vi "INI.GetPara.vi"(7 "section":string caption="Section", 8 "error in (no error)":errorcluster caption="错误输入（无错误）", 10 "Spec_name":string, 11 "INI_File":path) -> (0 "error out":errorcluster, 2 "Para out":string, 3 "ok?":bool)   [LabVIEW 2012, in "Lib_UEL.ATE.lvlib" / "Lib_App.lvlib"]
uses:
  Lib_App.lvlib
  <vilib>/Utility/config.llb/Read Key (String).vi
  <vilib>/Utility/config.llb/NI_LVConfig.lvlib
panel:
  # "说明:\n- 从配置文件读取参数."
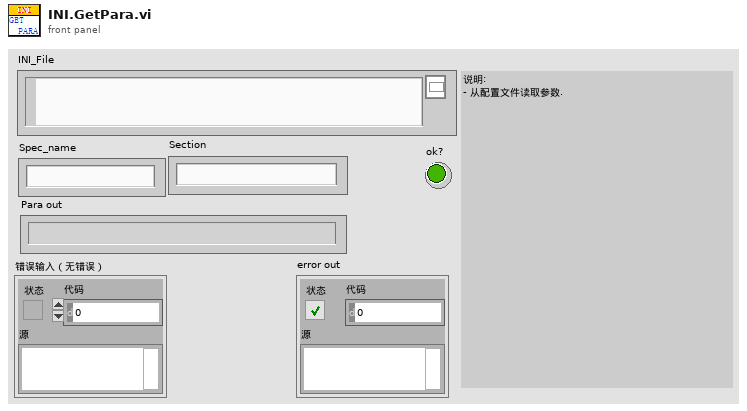
[diagram p1: front panel]
types:
  T1 = typedef "NI_LVConfig.lvlib/Config Data RefNum.ctl" = refnum<k1>
  T2 = cluster{"Item":string, "Unit":string, "Ref_value":dbl, "Low_limit_prod":dbl, "High_limit_prod":dbl, "Low_limit_qa":dbl, "High_limit_qa":dbl}
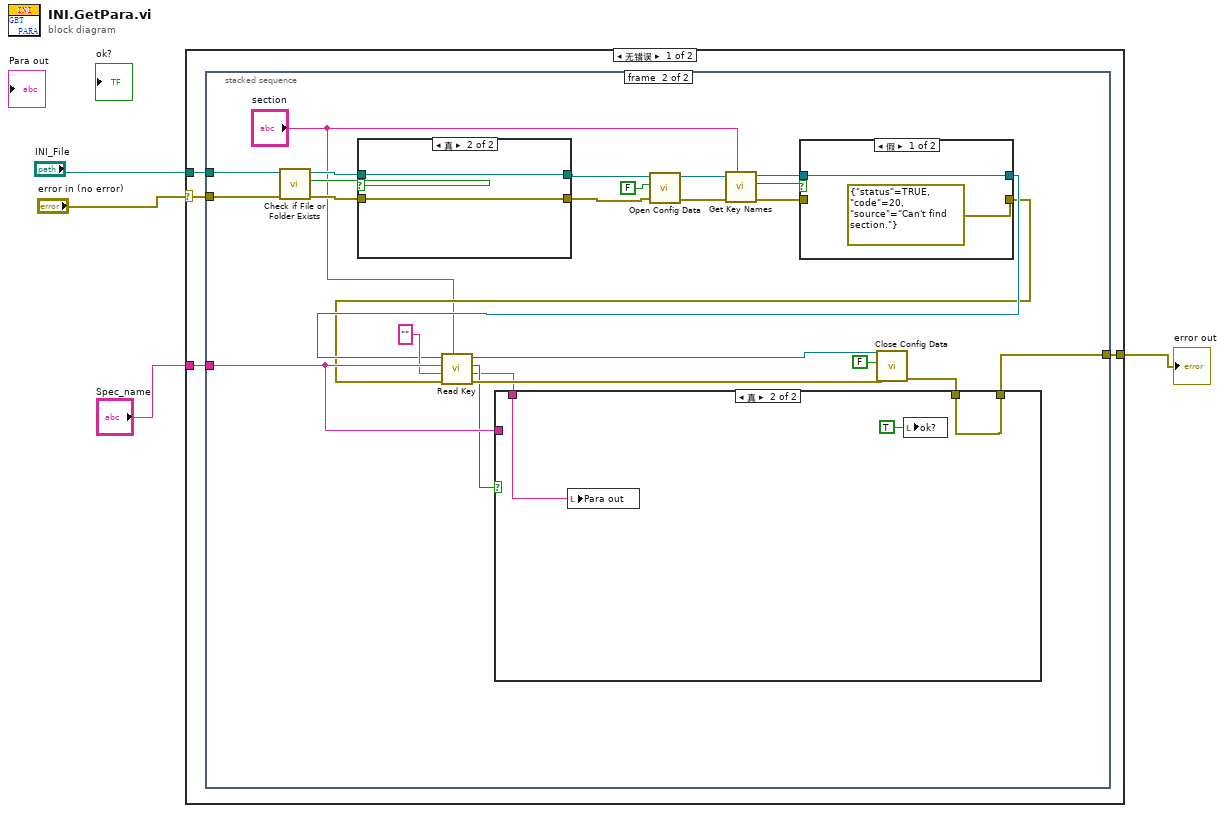
[diagram p0: block diagram]
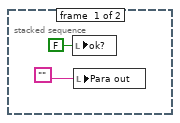
[diagram p2: hidden frame]
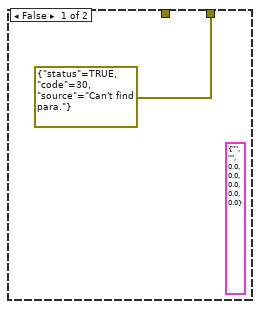
[diagram p3: hidden frame]
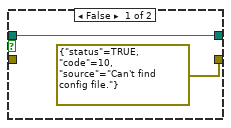
[diagram p5: hidden frame]
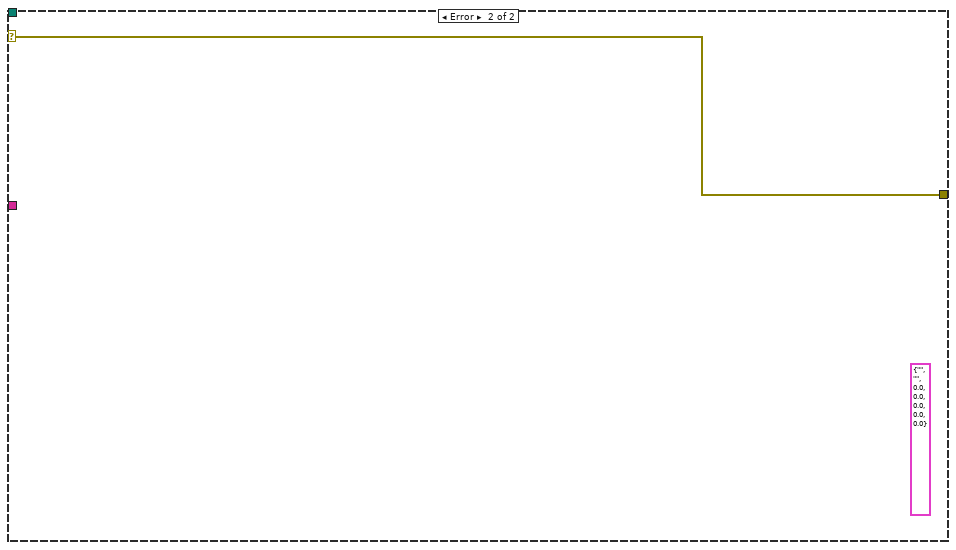
[diagram p6: hidden frame]
diagram:
  n1 = case shown="无错误" "error in (no error)" {
    selector: "error in (no error)" -> [w7 w48]
    tunnel: "INI_File" -> [w8 _]
    tunnel: [w6 w48] -> w2
    tunnel: "Spec_name" -> [w5 _]
    frame No Error {
      n2 = stacked-sequence {
        tunnel: w8 -> [_ w12]
        tunnel: w7 -> [_ w35]
        tunnel: [_ w33] -> w6
        tunnel: w5 -> [_ w34]
        frame #0 {
          n3 = local write "ok?"(FALSE ("ok?")) -> ()
          n4 = local write "Para out"("") -> ()
        }
        frame #1 {
          n5 = call <vilib>:"Check if File or Folder Exists.vi"("error in (no error)"=w35, "path"=w12) -> ("error out"=w30:errorcluster, "file or folder exists?"=w31:bool, "dup path"=w29:path)  [unwired: 7 in]
          n6 = case shown="真" w31 {
            tunnel: w30 -> [_ w46]
            tunnel: w29 -> [w45 w47]
            tunnel: [w45 w47] -> w28
            tunnel: [errorcluster {"status"=TRUE, "code"=10, "source"="Can't find config file."} ("error out") w46] -> w27
            frame False {
            }
            frame True {
            }
          }
          n7 = call <vilib>:"Open Config Data.vi"("error in (no error)"=w27, "create file if necessary (T)"=FALSE ("create file if necessary? (T)"), "configuration file path"=w28) -> ("error out"=w26:errorcluster, "refnum"=w25:T1)  [unwired: 6 in, 1 out]
          n8 = call <vilib>:"Get Key Names.vi"("section"="section", "error in (no error)"=w26, "refnum"=w25) -> ("error out"=w22:errorcluster, "section exists?"=w24:bool, "refnum out"=w23:T1)  [unwired: 5 in, 1 out]
          n9 = case shown="假" w24 {
            tunnel: w22 -> [_ w42]
            tunnel: w23 -> [w41 w43]
            tunnel: [w41 w43] -> w17
            tunnel: [errorcluster {"status"=TRUE, "code"=20, "source"="Can't find section."} ("error out") w42] -> w16
            frame False {
            }
            frame True {
            }
          }
          n10 = call-poly <vilib>:"Read Key.vi"("section"="section", "error in (no error)"=w16, "default value"="" ("section"), "key"=w34, "refnum"=w17) -> ("error out"=w20:errorcluster, "value"=w14:string, "found?"=w15:bool, "refnum out"=w21:T1)  [unwired: 3 in]
          n11 = call <vilib>:"Close Config Data.vi"("error in (no error)"=w20, "write file if changed (T)"=FALSE, "refnum"=w21) -> ("error out"=w13:errorcluster)  [unwired: 7 in, 1 out]
          n12 = case shown="真" w15 {
            tunnel: w14 -> [_ w37]
            tunnel: w13 -> [_ w39]
            tunnel: [errorcluster {"status"=TRUE, "code"=30, "source"="Can't find para."} ("error out") w39] -> w33
            tunnel: w34 -> [_ _]
            frame False {
              (unwired) T2 {"Item"="", "Unit"="", "Ref_value"=0.0, "Low_limit_prod"=0.0, "High_limit_prod"=0.0, "Low_limit_qa"=0.0, "High_limit_qa"=0.0} ("Spec")
            }
            frame True {
              n13 = local write "Para out"(w37) -> ()
              n14 = local write "ok?"(TRUE ("ok?")) -> ()
            }
          }
        }
      }
    }
    frame Error {
      (unwired) T2 {"Item"="", "Unit"="", "Ref_value"=0.0, "Low_limit_prod"=0.0, "High_limit_prod"=0.0, "Low_limit_qa"=0.0, "High_limit_qa"=0.0} ("Spec")
    }
  }
  "error out" <- w2
